vi "LJM get and check exp config.vi"(0 "Working Directory In":path, 1 "App Name":string) -> (4 "Write To File":bool, 6 "Data File Prefix":string="data", 7 "Interval (ms)":u32=500, 8 "Scan Rate (Hz)":dbl=500.0 format="%.3f", 10 "Graph History":i32=1000 min=0, 13 "Device Config File Name":string, 14 "Device Config Path":path, 15 "# Channels":i32=4, 16 "Disable Scaling":bool, 17 "Max File Size (Bytes)":i32=1048576, 18 "Channel Setup":T1={"+Ch"=["0", "1", "2", "3", "4", "5", "6", "7"], "-Ch"=["199", "199", "199", "199", "199", "199", "199", "199"], "Ranges"=[0, 0, 0, 0, 0, 0, 0, 0], "Scaling Equation"=["y=v0", "y=v1", "y=v2", "y=v3", "y=v4", "y=v5", "y=v6", "y=v7"], "Graph?"=[]} {"Ranges" items=["LJ_rgBIP10V", "LJ_rgBIP5V", "LJ_rgUNI5V", "LJ_rgUNI2P5V", "LJ_rgUNI1P25V", "LJ_rgBIP1V", "LJ_rgUNIP625V", "LJ_rgBIPP1V", "LJ_rgBIPP01V"]}, 19 "error out":errorcluster)   [LabVIEW 2022 SP3]
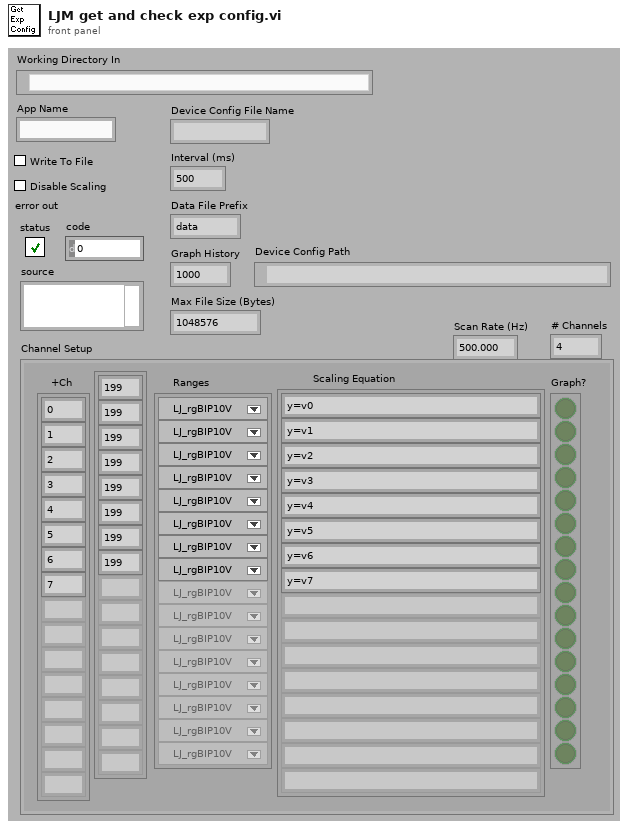
[diagram p1: front panel]
types:
  T1 = cluster{"+Ch":string[], "-Ch":string[], "Ranges":u16[], "Scaling Equation":string[], "Graph?":bool[]}
  T2 = enum16{"Left Button", "Center Button", "Right Button", "Window Close"}
  T3 = enum32{"existing file", "new file", "new or existing file", "existing dir", "new dir", "new or existing dir", "existing file (use LLBs)", "new file (use LLBs)", "new or existing file (use LLBs)", "new or existing file or directory (use LLBs)"}
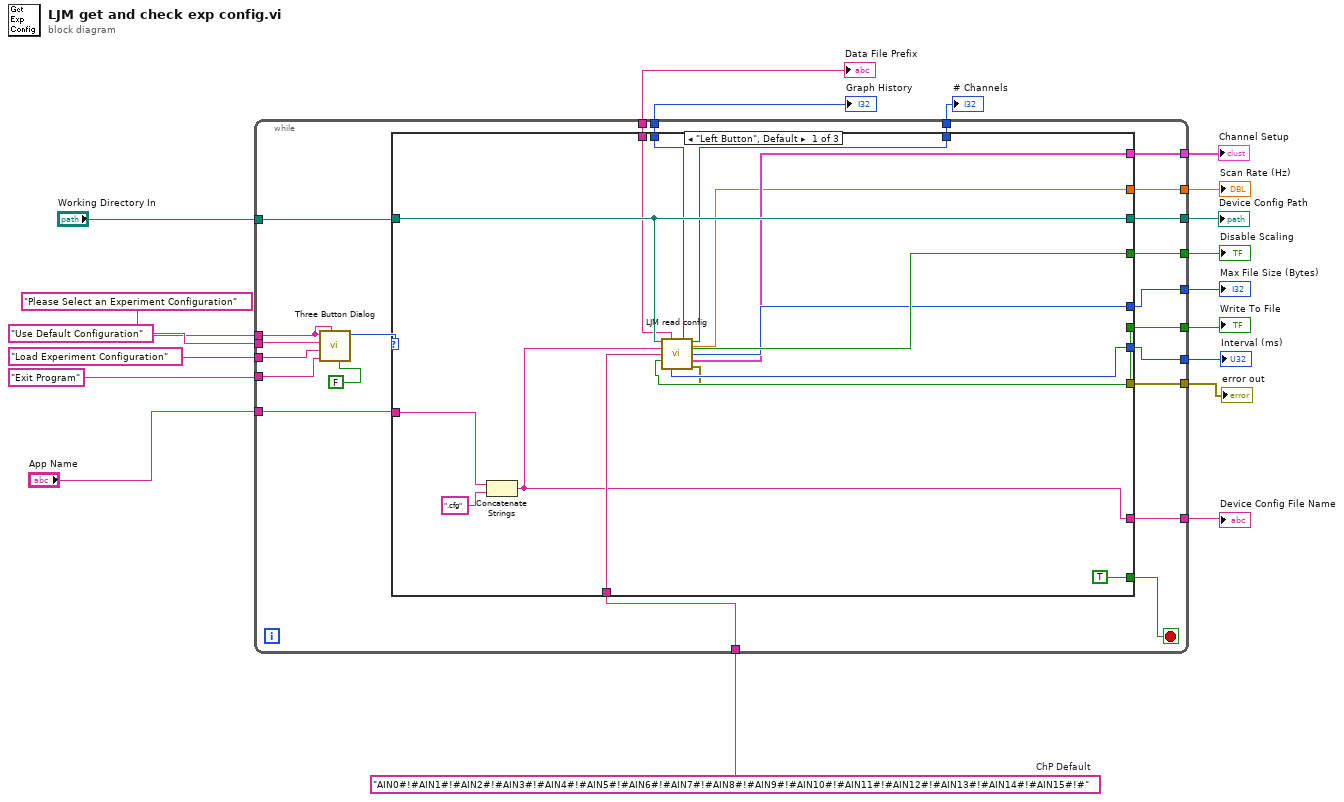
[diagram p0: block diagram]
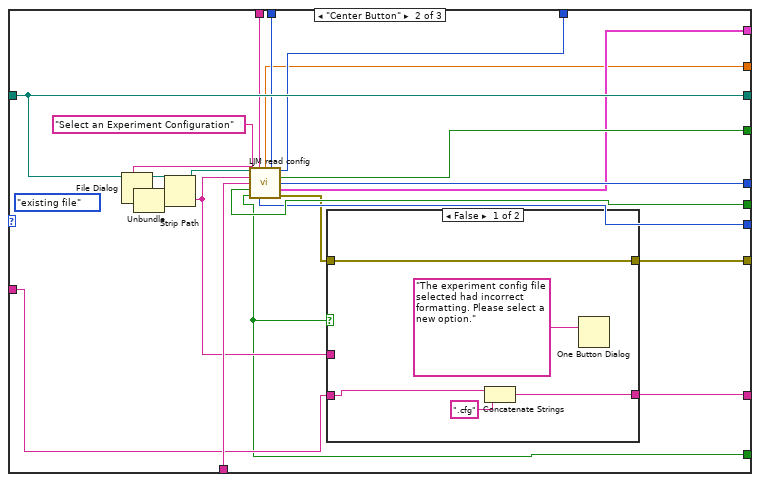
[diagram p2: hidden frame]
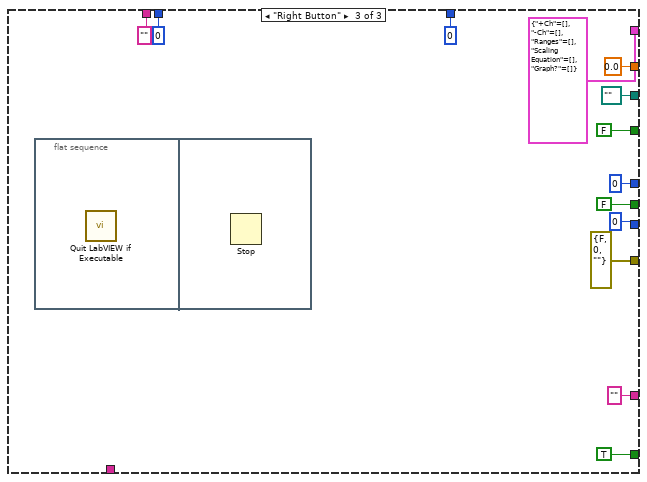
[diagram p4: hidden frame]
diagram:
  w5 = "AIN0#!#AIN1#!#AIN2#!#AIN3#!#AIN4#!#AIN5#!#AIN6#!#AIN7#!#AIN8#!#AIN9#!#AIN10#!#AIN11#!#AIN12#!#AIN13#!#AIN14#!#AIN15#!#"  # ChP Default
  n1 = while {
    tunnel: "Working Directory In" -> [w41]
    tunnel: "App Name" -> [w40]
    tunnel: [w39] -> w17
    tunnel: "Use Default Configuration" ("F button name (\"Cancel\")") -> [w24]
    tunnel: "Load Experiment Configuration" ("T button name (\"OK\")") -> [w38]
    tunnel: "Please Select an Experiment Configuration" ("message") -> [w22]
    tunnel: [w36] -> w13
    tunnel: [w35] -> w12
    tunnel: [w34] -> w11
    tunnel: [w33] -> w10
    tunnel: [w32] -> w9
    tunnel: [w31] -> w8
    tunnel: [w30] -> w7
    tunnel: [w29] -> w6
    tunnel: w5 -> [w28]
    tunnel: [w27] -> w4
    tunnel: [w26] -> w3
    tunnel: [w25] -> w2
    tunnel: "Exit Program" ("Right Button Text (\"Cancel\")") -> [w23]
    stop <- w20 stop-if-true
    n2 = call <vilib>:"Three Button Dialog.vi"("Allow user to close window? (TRUE)"=FALSE, "Window Title (\"\")"=w22, "Right Button Text (\"Cancel\")"=w23, "Center Button Text (\"No\")"=w38, "Left Button Text (\"Yes\")"=w24, "message"=w22) -> ("Which Button?"=w37:T2)  [unwired: 5 in]
    n3 = case shown="\"Left Button\", Default" w37 {
      tunnel: w41 -> [w55 w77 _]
      tunnel: w40 -> [w56 w64 _]
      tunnel: [w55 w77 path "" ("Working Directory In")] -> w39
      tunnel: [w54 w75 FALSE ("Write To File")] -> w36
      tunnel: [w53 w74 u32 0 ("Interval (ms)")] -> w35
      tunnel: [w51 w73 "" ("Data File Prefix")] -> w34
      tunnel: [w50 w72 0 ("Graph History")] -> w33
      tunnel: [w49 w71 0 ("# Channels")] -> w32
      tunnel: [w48 w70 FALSE ("Disable Scaling")] -> w31
      tunnel: [w47 w69 0 ("Max File Size (Bytes)")] -> w30
      tunnel: [w46 w68 T1 {"+Ch"=[], "-Ch"=[], "Ranges"=[], "Scaling Equation"=[], "Graph?"=[]} ("Channel Setup")] -> w29
      tunnel: w28 -> [w52 w67 _]
      tunnel: [w44 w63 "" ("name")] -> w27
      tunnel: [w45 w62 errorcluster {"status"=FALSE, "code"=0, "source"=""} ("error out")] -> w26
      tunnel: [w43 w60 0.0 ("Scan Rate (Hz)")] -> w25
      tunnel: [TRUE ("Good Experiment Config") w59 TRUE ("Good Experiment Config")] -> w20
      frame "Left Button", Default {
        n4 = Concatenate Strings(w56, ".cfg" ("filename")) -> (w44:string)
        n5 = call "LJM read config.vi"("Working Directory"=w55, "filename"=w44, "ChP Default"=w52) -> ("Data File Prefix"=w51:string, "Scan Rate (Hz)"=w43:dbl, "Graph History"=w50:i32, "# Channels"=w49:i32, "Disable Scaling"=w48:bool, "Max File Size (Bytes)"=w47:i32, "Write To File"=w54:bool, "Channel Setup"=w46:T1, "Interval (ms)"=w53:u32, "error out"=w45:errorcluster)  [unwired: 3 out]
      }
      frame "Center Button" {
        (unwired) T3."existing file" ("select mode (2)")
        n6 = File Dialog(7:"Select an Experiment Configuration" ("Substring"), 11:w77) -> (0:w58:errorcluster, 3:w76:path)  [unwired: 5 in, 2 out]
        n7 = Unbundle(w58) -> ()  [unwired: 3 out]
        n8 = Strip Path(path=w76) -> (stripped path=w61:path, name=w65:string)
        n9 = call "LJM read config.vi"("Working Directory"=w61, "filename"=w65, "ChP Default"=w67) -> ("Data File Prefix"=w73:string, "Scan Rate (Hz)"=w60:dbl, "Graph History"=w72:i32, "# Channels"=w71:i32, "Disable Scaling"=w70:bool, "Max File Size (Bytes)"=w69:i32, "Write To File"=w75:bool, "Channel Setup"=w68:T1, "Good Experiment Config"=w59:bool, "Interval (ms)"=w74:u32, "error out"=w66:errorcluster)  [unwired: 2 out]
        n10 = case shown="False" w59 {
          tunnel: w64 -> [w81 _]
          tunnel: [w80 w85] -> w63
          tunnel: w65 -> [_ w85]
          tunnel: w66 -> [w79 w84]
          tunnel: [w79 w84] -> w62
          frame False {
            n11 = Concatenate Strings(w81, ".cfg" ("string")) -> (w80:string)
            n12 = One Button Dialog(message="The experiment config file selected had incorrect formatting. Please select a new option.") -> ()  [unwired: 1 in, 1 out]
          }
          frame True {
          }
        }
      }
      frame "Right Button" {
        n13 = flat-sequence {
          frame #0 {
            n14 = call "Quit LabVIEW if Executable.vi"() -> ()  [unwired: 1 in]
          }
          frame #1 {
            n15 = Stop() -> ()  [unwired: 1 in]
          }
        }
      }
    }
  }
  "Device Config Path" <- w17
  "Device Config File Name" <- w4
  "error out" <- w3
  "Interval (ms)" <- w12
  "Write To File" <- w13
  "Data File Prefix" <- w11
  "Graph History" <- w10
  "# Channels" <- w9
  "Disable Scaling" <- w8
  "Max File Size (Bytes)" <- w7
  "Channel Setup" <- w6
  "Scan Rate (Hz)" <- w2
